vi "FTW-Scheduler-CheckShutdown.vi"(1 "FTW Job Scheduler":refnum<class "FTW-Scheduler.lvclass">) -> (0 "Shutdown?":bool)   [LabVIEW 2015, in "FTW-Scheduler.lvclass"]
uses:
  FTW-Scheduler.lvclass
  FTW-Scheduler.lvclass/FTW-Scheduler.ctl
panel:
  # "Inputs"
  # "Outputs"
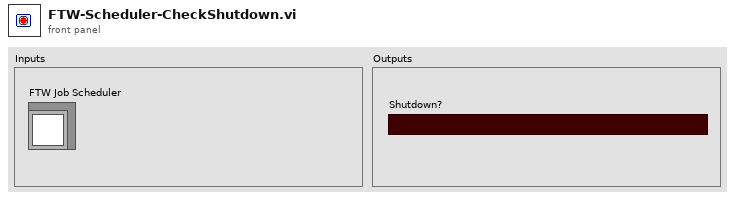
[diagram p1: front panel]
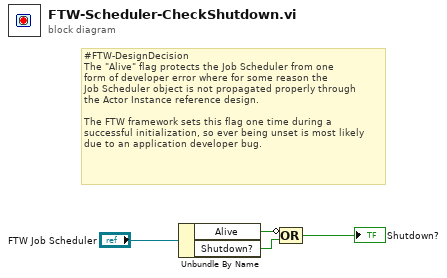
[diagram p0: block diagram]
diagram:
  # "#FTW-DesignDecision\nThe \"Alive\" flag protects the Job Scheduler from one\nform of developer error where for some reason the\nJob Scheduler object is not propagated properly through\nthe Actor Instance reference design.\n\nThe FTW framework sets this flag one time during a\nsuccessful initialization, so ever being unset is most likely\ndue to an application developer bug."
  n1 = Unbundle By Name("FTW Job Scheduler") -> ("Alive"=w3:bool, "Shutdown?"=w2:bool)
  n2 = Compound Arithmetic op=OR(invert w3, w2) -> (→"Shutdown?":bool)
